vi "ControlsVisibility.vi"(2 "Visible":bool, 3 "Array":refnum<vi>[](array[refnum])) -> ()   [LabVIEW 2019, in "ByteLVDevEnv.lvlib"]
uses:
  ByteLVDevEnv.lvlib
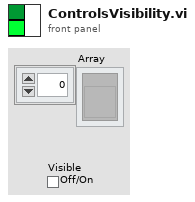
[diagram p1: front panel]
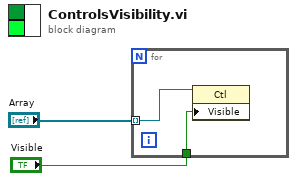
[diagram p0: block diagram]
diagram:
  n1 = for {
    tunnel: "Array" -> [w4] mode=indexing
    tunnel: "Visible" -> [w3]
    n2 = property class="Ctl"(reference=w4, "Visible"=w3) -> ()  [unwired: 1 in, 2 out]
  }
